vi "SLL DE AO LV2 Global Wrapper.vi"(4 "Wait for Response?":bool, 5 "Timeout (Sec)":dbl=5.0, 6 "AO value Array":dbl[](array[numeric]), 7 "AO Option":T2, 8 "error in (no error)":errorcluster, 9 "AO value":dbl, 10 "AO Channel Name Array":T1[](array[typedef]), 11 "AO Channel Name":T1) -> (0 "error out":errorcluster, 1 "Analog Output Array Value":dbl[](array[numeric]), 2 "Analog Output Line Value":dbl, 3 "Done?":bool)   [LabVIEW 2013]
uses:
  Controls/SLL DE AO Global Options.ctl
  Controls/SLL DE List of Analog Outputs.ctl
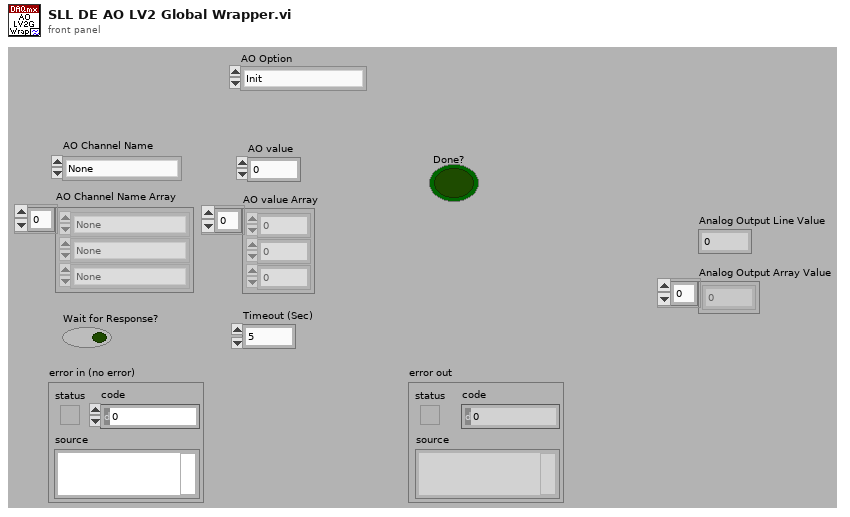
[diagram p1: front panel]
types:
  T1 = typedef "SLL DE List of Analog Outputs.ctl" = enum16{"None"}
  T2 = typedef "SLL DE AO Global Options.ctl" = enum16{"Init", "Write Line", "Write Array", "Read Line", "Read Array", "Read Full Status", "Restart AO", "Send to Safe Mode", "Stop AO"}
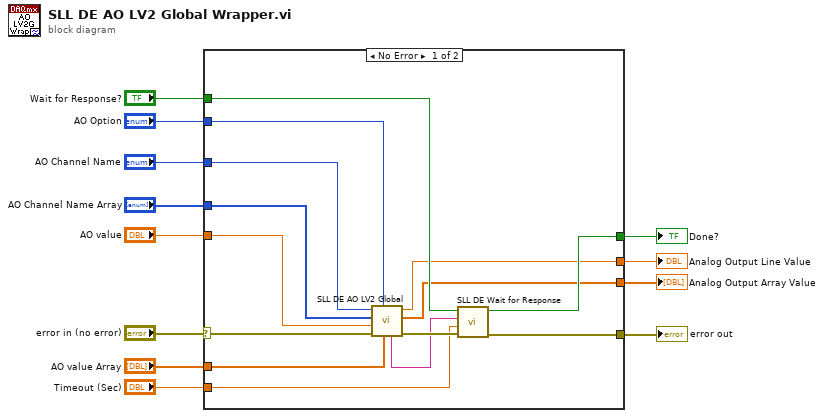
[diagram p0: block diagram]
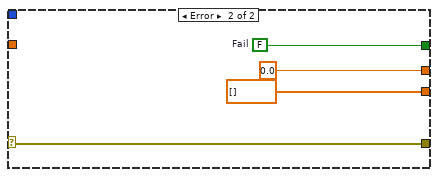
[diagram p2: hidden frame]
diagram:
  n1 = case shown="No Error" "error in (no error)" {
    selector: "error in (no error)" -> [w16 w30]
    tunnel: [w25 w30] -> w11
    tunnel: "AO Option" -> [w24 _]
    tunnel: "AO Channel Name" -> [w23 _]
    tunnel: "AO Channel Name Array" -> [w22 _]
    tunnel: "AO value" -> [w21 _]
    tunnel: "AO value Array" -> [w20 _]
    tunnel: "Wait for Response?" -> [w18 _]
    tunnel: [w17 w29] -> w4
    tunnel: [w15 0.0 ("Analog Output Line Value")] -> w3
    tunnel: [w14 dbl[] [] ("Analog Output Array Value")] -> w2
    tunnel: "Timeout (Sec)" -> [w13 _]
    frame No Error {
      n2 = call "SLL DE AO LV2 Global.vi"("AO value Array"=w20, "AO Option"=w24, "error in (no error)"=w16, "AO value"=w21, "AO Channel Name Array"=w22, "AO Channel Name"=w23) -> ("error out"=w26:errorcluster, "Analog Output Array Value"=w14:dbl[], "Analog Output Line Value"=w15:dbl, "Element Wrote"=w19:string)  [unwired: 2 in]
      n3 = call "SLL DE Wait for Response.vi"("Error In"=w26, "Timeout (Sec)"=w13, "Executed For?"=w19, "Check Response?"=w18) -> ("error out"=w25:errorcluster, "Done?"=w17:bool)  [unwired: 6 in]
    }
    frame Error {
      w29 = FALSE  # Fail
    }
  }
  "error out" <- w11
  "Done?" <- w4
  "Analog Output Line Value" <- w3
  "Analog Output Array Value" <- w2
